vi "Close Port.vi"(8 "error in (no error)":errorcluster, 11 "UART Actor in":refnum<class "UART Actor.lvclass">) -> (0 "error out":errorcluster, 3 "UART Actor out":refnum<class "UART Actor.lvclass">)   [LabVIEW 2020, in "UART Actor.lvlib" / "UART Actor.lvclass"]
uses:
  UART Actor.lvclass
  UART Actor.lvclass/UART Actor.ctl
  <vilib>/ActorFramework/Time-Delayed Send Message/Time-Delay Override Options.ctl
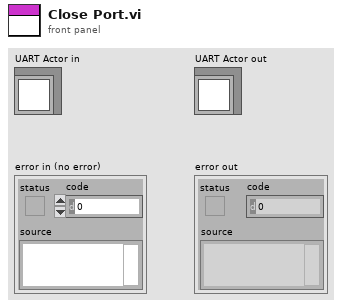
[diagram p1: front panel]
types:
  T1 = typedef "Time-Delay Override Options.ctl" = enum16{"Send next copy now", "Skip next scheduled copy", "Send next copy now and stop all further copies", "Stop all further copies"}
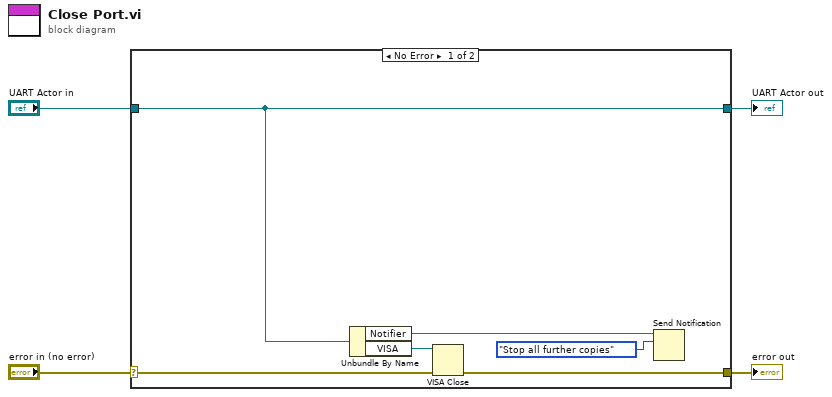
[diagram p0: block diagram]
diagram:
  n1 = case shown="No Error" "error in (no error)" {
    selector: "error in (no error)" -> [w10 w12]
    tunnel: [w8 w12] -> w3
    tunnel: [w9 w11] -> w1
    tunnel: "UART Actor in" -> [w9 w11]
    frame No Error {
      n2 = Unbundle By Name(w9) -> ("Notifier"=w6:refnum<notifier>, "VISA"=w7:refnum<visa-resource-name>)
      n3 = VISA Close(VISA resource name=w7, error in (no error)=w10) -> (error out=w8:errorcluster)
      n4 = Send Notification(notification=Time-Delay_Override_Options."Stop all further copies", notifier=w6) -> ()  [unwired: 1 in, 2 out]
    }
    frame Error {
    }
  }
  "error out" <- w3
  "UART Actor out" <- w1
